vi "inline wait.vi"(2 "ms wait":u32, 5 "error in (no error)":errorcluster) -> (4 "error out":errorcluster)   [LabVIEW 2016]
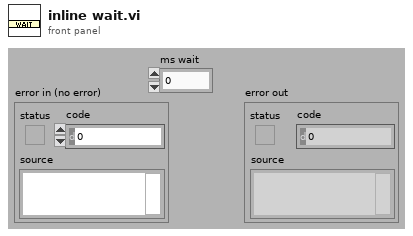
[diagram p1: front panel]
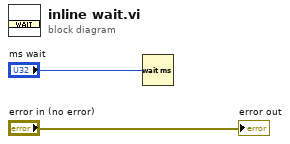
[diagram p0: block diagram]
diagram:
  n1 = Wait (ms)(milliseconds to wait="ms wait") -> ()  [unwired: 1 out]
  "error out" <- "error in (no error)"
